vi "Main.vi"() -> ()   [LabVIEW 2013]
uses:
  Control/State (State).ctl
  <vilib>/LabVIEW Interface for Arduino/LabVIEW Interface for Arduino.lvlib
  <vilib>/userdefined/High Color/IMAQdx.ctl
panel:
  out "error out":errorcluster
  in  "Camera":T1
  out "Tube":u8[][](graph)
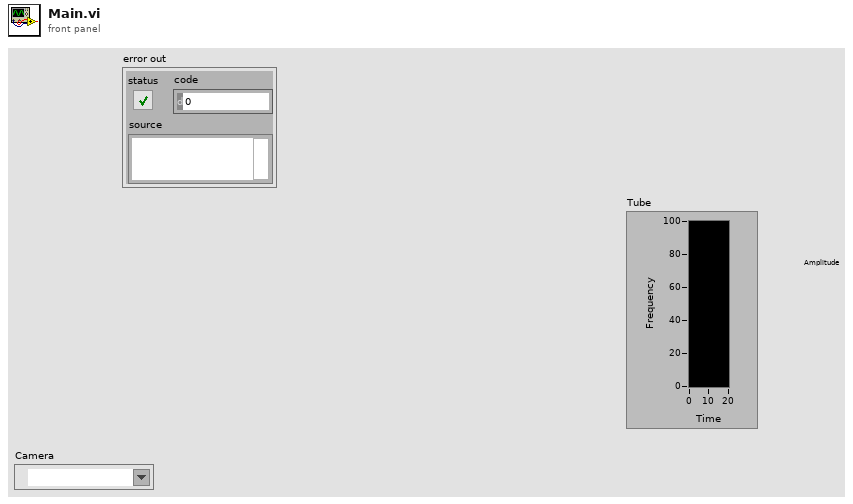
[diagram p1: front panel]
types:
  T1 = typedef "IMAQdx.ctl" = refnum<k21>
  T2 = typedef "State (State).ctl" = enum16{"Blank", "Init HW", "Start", "No pipes", "Pipes", "Quit", "Error"}
  T3 = typedef "IMAQ Image.ctl" = refnum<image>
  T4 = typedef "LabVIEW Interface for Arduino.lvlib/Arduino Resource.ctl" = cluster{"VISA resource":refnum<visa-resource-name>, "Board Type":T5, "Connection Type":enum8{"USB / Serial"}, "Bytes Per Packet (15)":u8}
  T5 = typedef "LabVIEW Interface for Arduino.lvlib/Board Type.ctl" = enum16{"Uno", "Dimuelanove w/Atmega 328", "Mega 2560"}
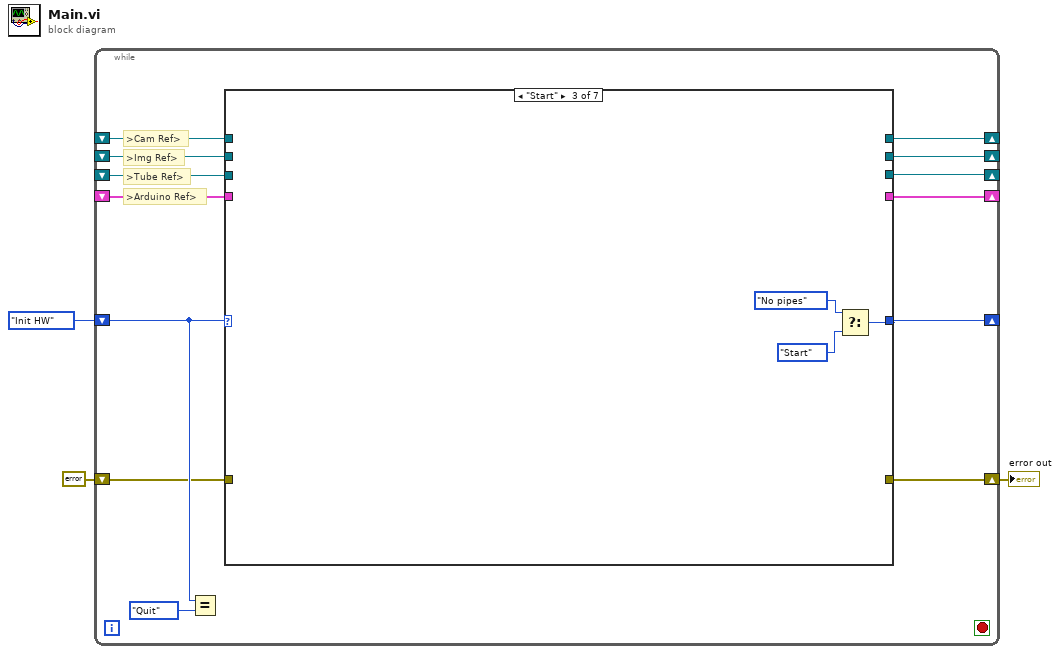
[diagram p0: block diagram]
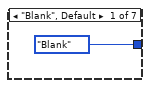
[diagram p2: hidden frame]
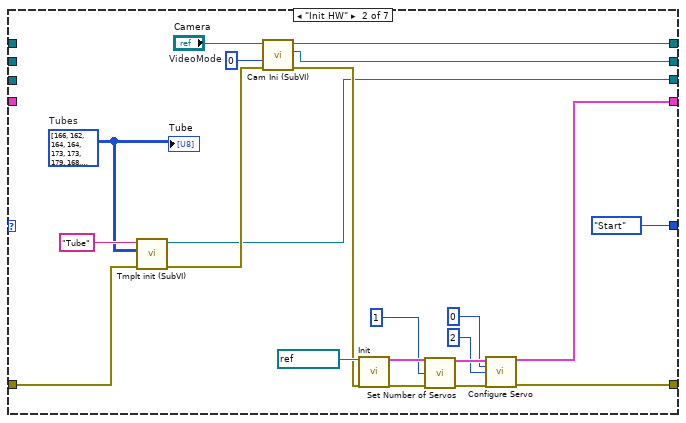
[diagram p3: hidden frame]
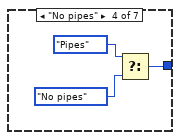
[diagram p4: hidden frame]
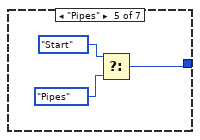
[diagram p5: hidden frame]
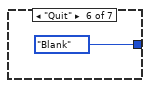
[diagram p6: hidden frame]
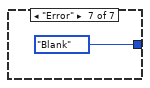
[diagram p7: hidden frame]
diagram:
  n1 = while {
    shift-right: [w16] -> _
    shift-left: State_(State)."Init HW" ("state") -> [w15]
    shift-right: [w13] -> w1
    shift-left: errorcluster {"status"=FALSE, "code"=0, "source"=""} ("error out") -> [w12]
    shift-right: [w11] -> _
    shift-left: _ -> [w10]
    shift-right: [w9] -> _
    shift-left: _ -> [w8]
    shift-right: [w7] -> _
    shift-left: _ -> [w6]
    shift-right: [w5] -> _
    shift-left: _ -> [w4]
    stop <- _ stop-if-true
    # ">Arduino Ref>"
    # ">Tube Ref>"
    # ">Img Ref>"
    # ">Cam Ref>"
    n2 = Equal?(x=w15, y=State_(State)."Quit") -> ()  [unwired: 1 out]
    n3 = case shown="\"Start\"" w15 {
      tunnel: [State_(State)."Blank" ("state") State_(State)."Start" ("state") w41 w42 w45 State_(State)."Blank" ("state") State_(State)."Blank" ("state")] -> w16
      tunnel: [_ w26 _ _ _ _ _] -> w13
      tunnel: w12 -> [_ w22 _ _ _ _ _]
      tunnel: [_ w25 _ _ _ _ _] -> w11
      tunnel: w10 -> [_ _ _ _ _ _ _]
      tunnel: [_ w24 _ _ _ _ _] -> w9
      tunnel: w8 -> [_ _ _ _ _ _ _]
      tunnel: [_ w20 _ _ _ _ _] -> w7
      tunnel: w6 -> [_ _ _ _ _ _ _]
      tunnel: [_ w18 _ _ _ _ _] -> w5
      tunnel: w4 -> [_ _ _ _ _ _ _]
      frame "Blank", Default {
      }
      frame "Init HW" {
        w19 = u8[][] [[166, 162, 164, 164, 173, 173, 179, 168, 212, 217, 232, 233, 234, 244, 255, 255, 255, 255, 255, 255, 255, 255, 255, 255, 255, 255, 255, 255, 255, 255, 243, 230, 223, 219, 217, 216, 218, 218, 219, 221, 218, 218, 218, 218, 221, 222, 220, 220, 217, 217, 222, 223, 218, 219, 223, 223, 217, 215, 220, 221, 218, 213, 227, 227, 218, 221, 215, 212, 217, 220, 213, 212, 212, 213, 215, 216, 215, 216, 221, 221, 215, 213, 214, 213, 206, 204, 209, 209, 208, 209, 205, 208, 208, 206, 206, 205, 211, 215, 207, 207], [146, 143, 144, 143, 143, 141, 154, 143, 205, 207, 222, 217, 215, 224, 228, 239, 255, 255, 255, 255, 255, 255, 255, 255, 255, 255, 255, 255, 255, 255, 230, 219, 217, 217, 215, 213, 220, 220, 221, 223, 219, 220, 222, 222, 221, 222, 219, 218, 228, 228, 223, 226, 214, 216, 220, 220, 214, 213, 218, 218, 220, 220, 216, 219, 218, 222, 215, 215, 216, 217, 217, 221, 210, 209, 217, 219, 220, 220, 215, 217, 218, 216, 206, 204, 201, 202, 201, 201, 201, 197, 200, 199, 200, 197, 199, 201, 203, 204, 209, 210], [132, 132, 130, 128, 130, 127, 138, 125, 186, 186, 193, 190, 188, 206, 205, 220, 221, 225, 231, 230, 225, 225, 229, 221, 235, 235, 255, 255, 255, 249, 225, 221, 213, 215, 213, 212, 217, 216, 212, 215, 225, 221, 217, 217, 221, 223, 215, 217, 220, 219, 220, 220, 218, 218, 217, 215, 223, 223, 224, 223, 214, 214, 215, 215, 221, 225, 222, 226, 219, 220, 216, 218, 216, 217, 216, 217, 216, 217, 213, 213, 209, 202, 201, 203, 181, 181, 183, 183, 180, 179, 180, 179, 179, 173, 177, 174, 193, 195, 191, 189], [122, 120, 121, 120, 122, 118, 127, 121, 156, 157, 153, 150, 143, 164, 178, 201, 198, 197, 203, 203, 201, 200, 196, 182, 212, 207, 255, 255, 254, 241, 223, 221, 215, 215, 218, 220, 215, 212, 214, 214, 215, 215, 220, 219, 221, 221, 227, 230, 219, 220, 217, 219, 221, 218, 220, 218, 219, 220, 220, 220, 217, 217, 217, 218, 220, 219, 217, 218, 216, 216, 220, 219, 218, 220, 213, 214, 214, 217, 219, 222, 211, 209, 189, 198, 169, 169, 171, 176, 170, 171, 172, 179, 171, 145, 143, 134, 159, 165, 183, 186], [110, 110, 115, 111, 112, 112, 111, 105, 128, 123, 123, 113, 110, 159, 163, 187, 198, 201, 196, 194, 200, 199, 185, 159, 188, 173, 250, 251, 249, 236, 223, 219, 222, 222, 221, 222, 217, 217, 217, 216, 215, 215, 223, 225, 215, 212, 217, 217, 224, 226, 214, 213, 216, 213, 214, 216, 214, 210, 218, 218, 219, 218, 219, 215, 219, 219, 221, 220, 221, 220, 218, 218, 211, 213, 213, 212, 221, 221, 221, 221, 206, 204, 177, 195, 170, 174, 166, 176, 181, 184, 175, 180, 163, 147, 125, 102, 133, 142, 145, 145], [109, 111, 109, 109, 111, 111, 117, 101, 111, 108, 99, 82, 104, 128, 166, 199, 198, 198, 198, 198, 199, 198, 187, 163, 185, 165, 246, 251, 255, 240, 222, 218, 219, 218, 222, 222, 220, 219, 220, 220, 217, 216, 219, 219, 221, 221, 220, 220, 220, 220, 222, 220, 221, 218, 222, 221, 221, 222, 215, 210, 214, 214, 213, 210, 213, 213, 215, 215, 218, 220, 213, 215, 210, 211, 216, 216, 213, 216, 217, 217, 201, 202, 188, 198, 172, 196, 183, 185, 186, 183, 190, 183, 177, 149, 116, 81, 110, 122, 123, 125], [132, 130, 125, 125, 128, 125, 130, 127, 120, 106, 83, 72, 101, 143, 174, 212, 202, 202, 207, 206, 209, 208, 197, 154, 187, 162, 255, 255, 255, 251, 238, 231, 222, 223, 218, 221, 215, 217, 215, 214, 221, 221, 216, 217, 222, 221, 220, 216, 218, 218, 212, 215, 222, 221, 219, 219, 218, 218, 218, 218, 214, 217, 216, 216, 217, 219, 210, 215, 214, 217, 212, 211, 214, 214, 218, 217, 217, 220, 219, 221, 208, 206, 180, 219, 194, 209, 194, 199, 194, 194, 192, 192, 177, 150, 115, 74, 96, 116, 119, 124], [145, 145, 143, 140, 143, 138, 137, 137, 137, 112, 94, 60, 91, 130, 175, 203, 219, 219, 213, 213, 219, 219, 207, 167, 186, 159, 255, 255, 255, 255, 255, 243, 218, 217, 210, 211, 217, 221, 217, 214, 220, 219, 214, 213, 218, 220, 217, 214, 219, 216, 217, 214, 220, 220, 216, 215, 216, 216, 216, 215, 221, 221, 216, 215, 214, 213, 216, 212, 220, 222, 215, 216, 217, 217, 215, 218, 215, 215, 213, 212, 207, 207, 184, 217, 198, 207, 200, 200, 206, 207, 208, 208, 185, 141, 111, 70, 88, 116, 126, 125], [155, 156, 150, 150, 157, 156, 153, 154, 147, 129, 101, 74, 104, 146, 184, 203, 211, 211, 213, 213, 217, 217, 210, 170, 189, 160, 254, 255, 255, 255, 255, 255, 232, 221, 219, 219, 220, 221, 216, 217, 218, 218, 221, 222, 213, 212, 217, 219, 219, 218, 220, 219, 217, 217, 219, 221, 217, 216, 220, 219, 215, 214, 218, 218, 216, 217, 212, 211, 213, 214, 214, 212, 214, 214, 213, 217, 216, 217, 220, 221, 202, 199, 184, 212, 199, 208, 203, 202, 205, 205, 211, 210, 177, 140, 107, 70, 99, 126, 130, 140], [167, 167, 166, 164, 167, 168, 168, 170, 167, 136, 112, 72, 96, 129, 166, 199, 211, 211, 211, 211, 209, 209, 204, 179, 188, 159, 255, 255, 255, 255, 255, 255, 238, 228, 223, 221, 223, 220, 219, 217, 219, 219, 217, 217, 213, 214, 215, 216, 221, 222, 216, 216, 218, 214, 221, 221, 214, 214, 218, 218, 214, 212, 220, 219, 210, 208, 215, 215, 215, 215, 215, 214, 212, 213, 209, 211, 215, 215, 219, 221, 207, 204, 188, 224, 196, 207, 207, 207, 200, 201, 204, 204, 190, 141, 107, 77, 99, 129, 148, 159], [182, 183, 182, 181, 176, 176, 178, 177, 169, 152, 120, 90, 103, 137, 171, 194, 194, 194, 196, 197, 201, 200, 199, 158, 190, 163, 255, 255, 255, 255, 255, 255, 255, 238, 220, 217, 220, 221, 218, 221, 217, 219, 217, 217, 216, 215, 219, 215, 218, 218, 222, 222, 221, 219, 218, 218, 216, 216, 219, 219, 216, 215, 210, 212, 211, 211, 212, 210, 216, 214, 215, 217, 216, 216, 214, 217, 215, 215, 218, 214, 203, 215, 190, 221, 203, 209, 200, 200, 206, 206, 201, 200, 178, 139, 100, 74, 117, 151, 160, 167], [184, 187, 193, 193, 187, 187, 189, 189, 181, 160, 134, 79, 108, 140, 161, 187, 189, 189, 185, 185, 192, 193, 191, 159, 192, 166, 255, 255, 255, 255, 255, 255, 255, 246, 226, 221, 214, 215, 223, 223, 215, 214, 221, 223, 212, 211, 214, 215, 213, 212, 216, 217, 219, 221, 215, 213, 215, 213, 216, 219, 215, 214, 215, 216, 217, 216, 221, 220, 214, 215, 208, 209, 216, 215, 212, 215, 208, 209, 215, 214, 206, 215, 185, 223, 195, 202, 189, 189, 184, 185, 187, 184, 166, 129, 96, 76, 124, 162, 172, 181], [196, 197, 201, 201, 202, 202, 202, 202, 193, 166, 136, 88, 96, 135, 151, 175, 180, 182, 184, 185, 175, 177, 182, 150, 182, 154, 255, 255, 255, 255, 255, 255, 255, 255, 236, 229, 220, 221, 220, 221, 217, 217, 213, 211, 222, 223, 219, 219, 212, 213, 219, 218, 219, 222, 221, 219, 218, 219, 219, 219, 221, 222, 221, 218, 214, 215, 212, 211, 216, 216, 215, 213, 215, 215, 217, 217, 213, 217, 218, 215, 200, 208, 189, 214, 191, 196, 183, 183, 178, 178, 176, 172, 157, 119, 99, 71, 130, 170, 180, 191], [196, 196, 202, 202, 204, 204, 204, 204, 196, 167, 135, 80, 98, 135, 146, 172, 171, 173, 169, 171, 175, 177, 170, 147, 179, 148, 255, 255, 255, 255, 255, 255, 255, 255, 236, 223, 217, 217, 225, 225, 212, 215, 219, 218, 213, 212, 219, 218, 215, 215, 218, 219, 214, 214, 217, 219, 214, 217, 216, 214, 219, 220, 215, 216, 215, 215, 213, 216, 214, 215, 213, 212, 214, 215, 209, 209, 219, 220, 213, 211, 201, 207, 186, 211, 185, 187, 173, 173, 179, 177, 170, 171, 159, 118, 92, 60, 132, 167, 182, 191], [188, 189, 198, 198, 206, 206, 194, 194, 183, 159, 124, 72, 91, 128, 146, 169, 160, 162, 160, 160, 160, 163, 167, 133, 180, 156, 255, 255, 255, 255, 255, 255, 255, 255, 243, 231, 217, 215, 215, 215, 219, 219, 215, 215, 217, 217, 216, 215, 220, 221, 214, 214, 219, 219, 214, 215, 215, 215, 215, 214, 218, 215, 217, 218, 211, 211, 216, 219, 212, 213, 216, 217, 214, 214, 213, 211, 217, 215, 208, 205, 198, 201, 183, 203, 176, 181, 164, 163, 166, 166, 160, 159, 138, 105, 89, 61, 131, 173, 187, 195]]  # Tubes
        w29 = u32 0  # VideoMode
        n4 = call "Tmplt init (SubVI).vi"("error in"=w22, "Template"=w19, "Image Name"="Tube") -> ("error out"=w21:errorcluster, "Image Out"=w20:T3)  [unwired: 7 in]
        n5 = call "Cam Ini (SubVI).vi"("error in"=w21, "VideoMode"=w29, "Camera"="Camera") -> ("error out"=w27:errorcluster, "Image Ref"=w24:T3, "Cam Ref"=w25:T1)  [unwired: 6 in]
        n6 = call <vilib>:"Init.vi"("VISA resource"=refnum<visa-resource-name> "COM3", "error in"=w27) -> ("Arduino Resource"=w37:T4, "error out"=w36:errorcluster)  [unwired: 16 in]
        n7 = call <vilib>:"Set Number of Servos.vi"("Arduino Resource"=w37, "Number Of Servos (1)"=u8 1, "error in"=w36) -> ("Arduino Resource"=w35:T4, "error out"=w34:errorcluster)  [unwired: 11 in]
        n8 = call <vilib>:"Configure Servo.vi"("Arduino Resource"=w35, "Servo Number (0)"=u8 0 ("Servo Number"), "DIO Pin (2)"=u8 2 ("Servo Number"), "error in"=w34) -> ("Arduino Resource"=w18:T4, "error out"=w26:errorcluster)  [unwired: 10 in]
        "Tube" <- w19
      }
      frame "Start" {
        n9 = Select(t=State_(State)."No pipes" ("state"), f=State_(State)."Start" ("state")) -> (s? t:f=w41:T2)  [unwired: 1 in]
      }
      frame "No pipes" {
        n10 = Select(t=State_(State)."Pipes" ("state"), f=State_(State)."No pipes" ("state")) -> (s? t:f=w42:T2)  [unwired: 1 in]
      }
      frame "Pipes" {
        n11 = Select(t=State_(State)."Start" ("state"), f=State_(State)."Pipes" ("state")) -> (s? t:f=w45:T2)  [unwired: 1 in]
      }
      frame "Quit" {
      }
      frame "Error" {
      }
    }
  }
  "error out" <- w1
